vi "LidarSetToContinousMeasurement.vi"(1 "SelectLIDAR":enum16{"Raphael", "Leonardo"}(ring)) -> ()   [LabVIEW 2010]
doc: "LidarSetToContinuousMeasurement.vi sends a command to the selected LIDAR to set it to continuously stream data,\n\n<b>Inputs</b>\nSelectLIDAR - selects which LIDAR to set to continuous measurement."
uses:
  <vilib>/rvi/DataTransferAndStorage/Container/XNode/niFpgaContainer.xnode
  <vilib>/rvi/DataTransferAndStorage/Container/Common/niFpgaTransferTypeControl.ctl
  <vilib>/rvi/FIFO/Fifo_Types/niFpgaFifoControlLogicControl.ctl
  <vilib>/rvi/DataTransferAndStorage/Container/Common/niFpgaContainerMethod.ctl
  <vilib>/rvi/DataTransferAndStorage/Container/Common/niFpgaContainerMetaDataKey.ctl
  <vilib>/rvi/DataTransferAndStorage/FIFO/niFpgaPeerToPeerStreamState.ctl
  <vilib>/rvi/DataTransferAndStorage/Container/Common/niFpgaContainerExecOnDevCompGetState.vi
  <vilib>/rvi/FIFO/Fifo_Resource/nirvififoEmulationSetSize.vi
  <vilib>/rvi/DataTransferAndStorage/Container/Common/niFpgaContainerGetUniqueNameForEmu.vi
  <vilib>/rvi/interface/RandomDataEmulation/nirviRandomDataFPGAFIFO.vi
  <vilib>/rvi/interface/RandomDataEmulation/niFpgaRandomDataHandleErrors.vi
  <vilib>/rvi/eio/common/nirviEmuReportErrorAndStop.vi
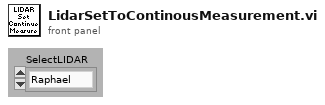
[diagram p1: front panel]
types:
  T1 = typedef "niFpgaFifoControlLogicControl.ctl" = enum16{"Slice Fabric", "Target Optimal", "Built-in"}
  T2 = typedef "niFpgaContainerMethod.ctl" = enum16{"<none>", "write", "read", "clear", "getNumberOfElementsToWrite", "getNumberOfElementsToRead", "enable", "disable", "flushAndDisable", "getStreamState", "readA", "readB", "dramWrite", "dramWriteWithByteEnables", "dramRequestData", "dramRetrieveData"}
  T3 = typedef "niFpgaTransferTypeControl.ctl" = enum16{"Target-Scoped", "Host to Target - DMA", "Target to Host - DMA", "Peer to Peer Reader", "Peer to Peer Writer", "Bidirectional"}
  T4 = typedef "niFpgaPeerToPeerStreamState.ctl" = enum16{"Unlinked", "Disabled", "Enabled", "Flushing"}
  T5 = typedef "niFpgaContainerMetaDataKey.ctl" = enum16{"FPGA FIFO", "FPGA Memory", "FPGA Register"}
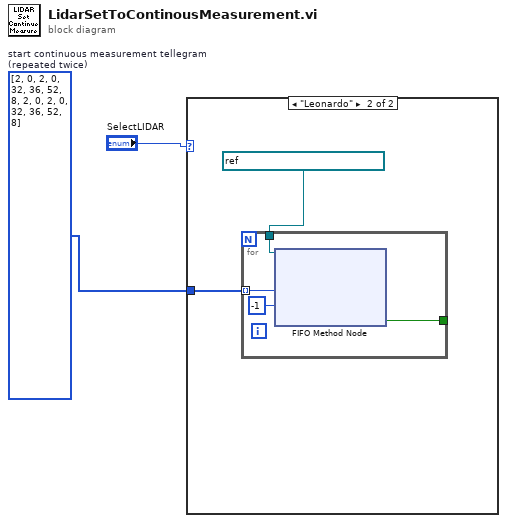
[diagram p0: block diagram]
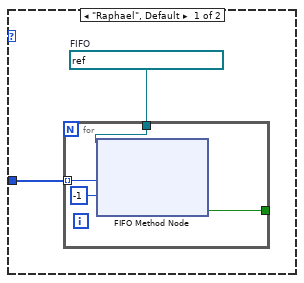
[diagram p2: hidden frame]
diagram:
  w2 = u8[] [2, 0, 2, 0, 32, 36, 52, 8, 2, 0, 2, 0, 32, 36, 52, 8]  # start continuous measurement tellegram (repeated twice)
  n1 = case shown="\"Leonardo\"" "SelectLIDAR" {
    tunnel: w2 -> [w4 w326]
    frame "Raphael", Default {
      w3 = refnum<k21> "LIDARRaphaelWriteFIFO"  # FIFO
      n2 = for {
        tunnel: w4 -> [w8] mode=indexing
        tunnel: [w6] -> _
        tunnel: w3 -> [w5]
        n3 = xnode ("FIFO Method Node")("Element"=w8, "Timeout"=-1, "FIFO In"=w5) -> ("Timed Out?"=w6:bool)  [unwired: 1 out]
      }
    }
    frame "Leonardo" {
      n4 = for {
        tunnel: w326 -> [w331] mode=indexing
        tunnel: [w329] -> _
        tunnel: refnum<k21> "LIDARLeonardoWriteFIFO" ("Write FIFO") -> [w328]
        n5 = xnode ("FIFO Method Node")("Element"=w331, "Timeout"=-1, "FIFO In"=w328) -> ("Timed Out?"=w329:bool)  [unwired: 1 out]
      }
    }
  }
